vi "FTW-Endpoint-Payload-Request-Receive.vi"(0 "FTW Endpoint":refnum<class "FTW-Endpoint-TCP.lvclass">, 5 "Timeout":i32 format="%dmsec", 11 "error in":errorcluster) -> (4 "FTW Endpoint out":refnum<class "FTW-Endpoint-TCP.lvclass">, 6 "Reply Endpoint":refnum<class "FTW-Endpoint.lvclass">, 8 "Payload":T1, 10 "Timed out?":bool, 15 "error out":errorcluster)   [LabVIEW 2013, in "FTW-Endpoint-TCP.lvclass"]
uses:
  FTW-Endpoint-TCP.lvclass
  Payload/FTW-MessagePayload.ctl
  Endpoint/FTW-Endpoint.lvclass
panel:
  # "Inputs"
  # "Outputs"
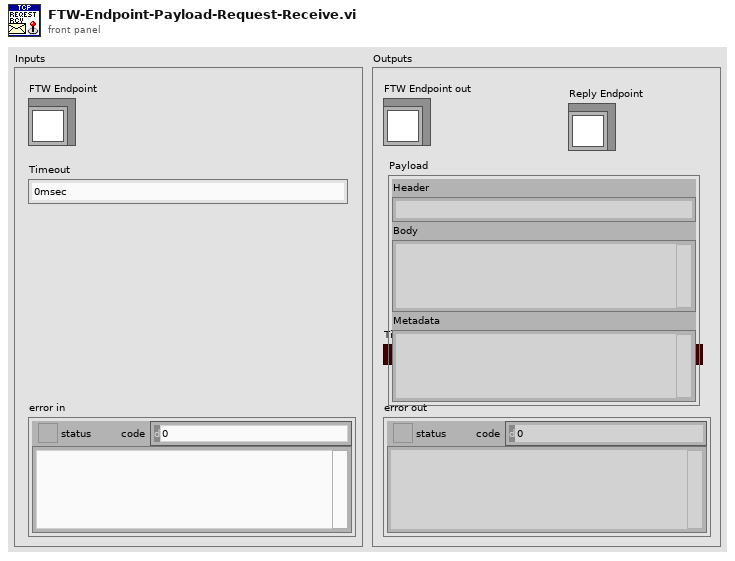
[diagram p1: front panel]
types:
  T1 = typedef "FTW-MessagePayload.ctl" = cluster{"Header":string, "Body":string, "Metadata":string}
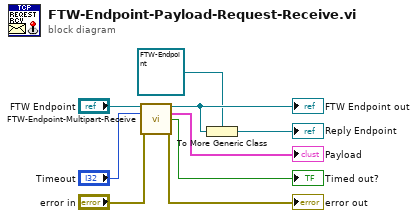
[diagram p0: block diagram]
diagram:
  n1 = call-dynamic "FTW-Endpoint-Multipart-Receive.vi"("FTW Endpoint"="FTW Endpoint", "Timeout"="Timeout", "error in"="error in") -> ("FTW Endpoint out"=w6:refnum<class "FTW-Endpoint-TCP.lvclass">, "Message Received"=→"Payload":T1, "Timed out?"=→"Timed out?":bool, "error out"=→"error out":errorcluster)  [unwired: 9 in]
  "FTW Endpoint out" <- w6
  n2 = To More Generic Class(target class=refnum<class "FTW-Endpoint.lvclass"> refnum ("FTW Endpoint"), reference=w6) -> (generic class reference=→"Reply Endpoint":refnum<class "FTW-Endpoint.lvclass">)
